vi "PLC控制写入.vi"(8 "error in (no error)":errorcluster caption="错误输入（无错误）", 10 "PLC指令":T2={"变量类型"=2, "PLC地址"=0, "size"=0, "写入数据(写入时有效)"=0} {"变量类型" items=["X", "Y", "M", "D"]}, 11 "PLC设置":T1) -> (0 "error out":errorcluster caption="错误输出", 2 "返回值":i32, 3 "PLC设置2":T1)   [LabVIEW 2015, in "Action.lvlib"]
uses:
  Action.lvlib
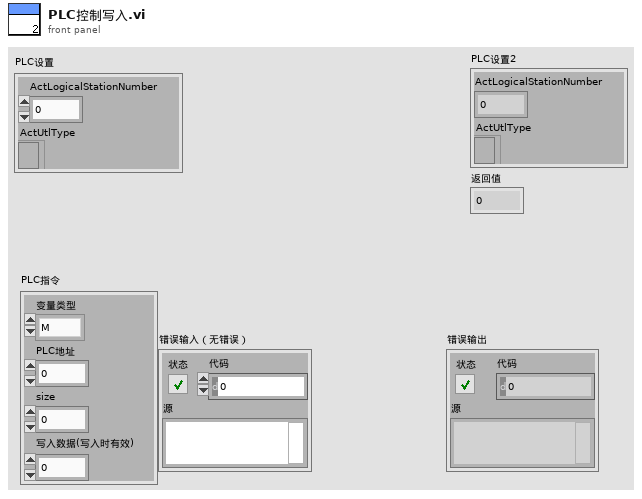
[diagram p1: front panel]
types:
  T1 = typedef "Action.lvlib/PLC设置.ctl" = cluster{"ActLogicalStationNumber":i32, "ActUtlType":refnum<k7>}
  T2 = typedef "Action.lvlib/PLC控制指令.ctl" = cluster{"变量类型":u32, "PLC地址":i32, "size":i32, "写入数据(写入时有效)":i16}
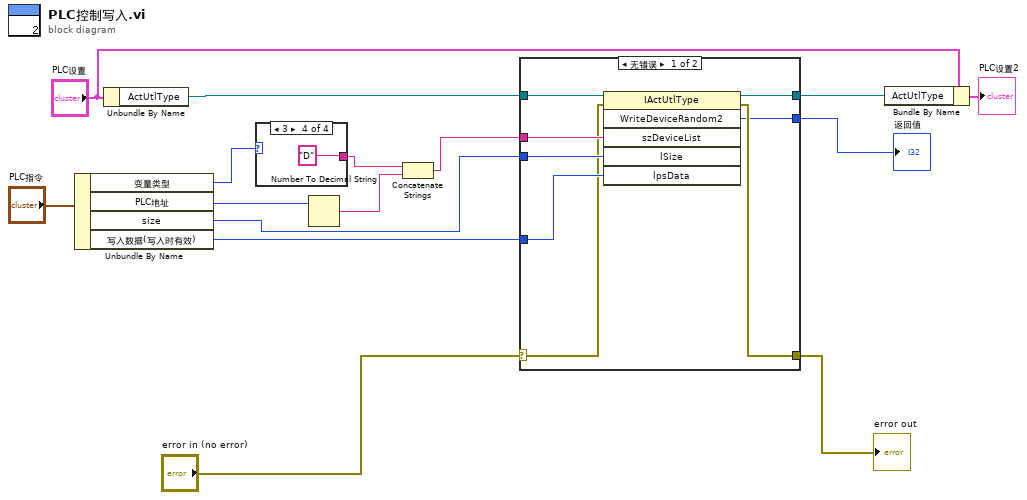
[diagram p0: block diagram]
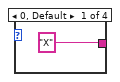
[diagram p2: hidden frame]
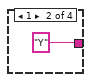
[diagram p3: hidden frame]
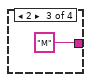
[diagram p4: hidden frame]
diagram:
  n1 = Unbundle By Name("PLC指令") -> ("变量类型"=w11:u32, "PLC地址"=w9:i32, "size"=w6:i32, "写入数据(写入时有效)"=w5:i16)
  n2 = Unbundle By Name("PLC设置") -> ("ActUtlType"=w12:refnum<k7>)
  n3 = case shown="3" w11 {
    tunnel: ["X" "Y" "M" "D"] -> w10
    frame 0, Default {
    }
    frame 1 {
    }
    frame 2 {
    }
    frame 3 {
    }
  }
  n4 = Number To Decimal String(number=w9) -> (decimal integer string=w8:string)  [unwired: 1 in]
  n5 = Concatenate Strings(w10, w8) -> (w7:string)
  n6 = case shown="无错误" "error in (no error)" {
    selector: "error in (no error)" -> [w22 w29]
    tunnel: [w21 w29] -> w13
    tunnel: w12 -> [w27 w28]
    tunnel: w7 -> [w26 _]
    tunnel: w6 -> [w25 _]
    tunnel: w5 -> [w24 _]
    tunnel: [w23 w28] -> w3
    tunnel: [w20 _] -> w1
    frame No Error {
      n7 = invoke class="IActUtlType" method="WriteDeviceRandom2"(reference=w27, error in=w22, "szDeviceList"=w26, "lSize"=w25, "lpsData"=w24) -> (reference out=w23:refnum<k7>, error out=w21:errorcluster, "WriteDeviceRandom2"=w20:i32)  [unwired: 1 in, 3 out]
    }
    frame Error {
    }
  }
  "error out" <- w13
  "返回值" <- w1
  n8 = Bundle By Name(cluster="PLC设置", "ActUtlType"=w3) -> (→"PLC设置2":T1)
